vi "ziSetValueComplex.vi"(3 "Error In":errorcluster, 4 "Value":cdb, 5 "Path":string, 6 "Handle In":T1 {"Handle" format="0x%08x"; "Conn" format="0x%08x"}) -> (0 "Error Out":errorcluster, 2 "Handle Out":T1 {"Handle" format="0x%08x"; "Conn" format="0x%08x"})   [LabVIEW 2018, in "Zurich Instruments LabOne.lvlib"]
doc: "This vi sets values to the nodes specified in Path to Value. More than one node can be set if a wildcard is used in Path."
uses:
  Zurich Instruments LabOne.lvlib
  <instrlib>/Zurich Instruments LabOne/Private/ziLV64.framework
  ziTypeHandle.ctl
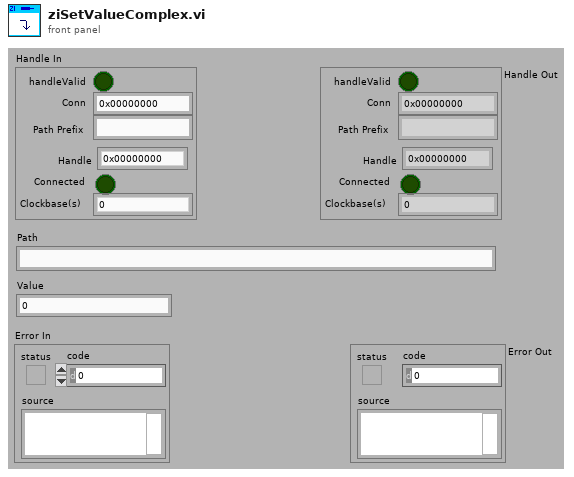
[diagram p1: front panel]
types:
  T1 = typedef "Zurich Instruments LabOne.lvlib/ziTypeHandle.ctl" = cluster{"handleValid":bool, "Conn":u64, "Path Prefix":string, "Handle":u64, "Connected":bool, "Clockbase(s)":dbl}
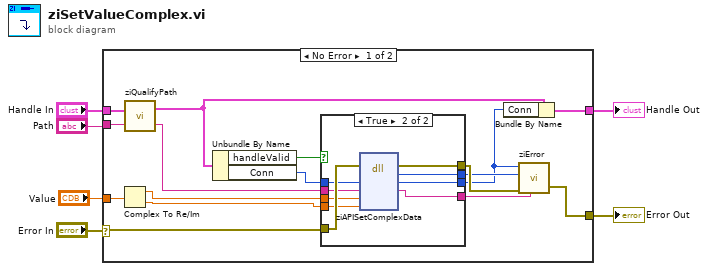
[diagram p0: block diagram]
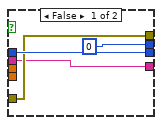
[diagram p2: hidden frame]
diagram:
  n1 = case shown="No Error" "Error In" {
    selector: "Error In" -> [w11 w37]
    tunnel: "Value" -> [w9 _]
    tunnel: [w21 w37] -> w5
    tunnel: [w17 w36] -> w4
    tunnel: "Handle In" -> [w16 w36]
    tunnel: "Path" -> [w14 _]
    frame No Error {
      n2 = Complex To Re/Im(x + iy=w9) -> (x=w8:dbl, y=w7:dbl)
      n3 = call "ziQualifyPath.vi"("Path In"=w14, "Handle In"=w16) -> ("Path Out"=w13:string, "Handle Out"=w15:T1)
      n4 = Unbundle By Name(w15) -> ("handleValid"=w18:bool, "Conn"=w22:u64)
      n5 = case shown="True" w18 {
        tunnel: w11 -> [w25 w35]
        tunnel: w22 -> [w26 w34]
        tunnel: w13 -> [w23 w33]
        tunnel: w8 -> [_ w32]
        tunnel: [w25 w31] -> w20
        tunnel: [u32 0 ("return type") w30] -> w19
        tunnel: [w26 w29] -> w10
        tunnel: [w23 w28] -> w12
        tunnel: w7 -> [_ w27]
        frame False {
        }
        frame True {
          n6 = dll-call lib="Applications/National Instruments/LabVIEW 2019 64-bit/instr.lib/Zurich Instruments LabOne/Private/ziLV*.*" fn="ziAPISetComplexData"(error in=w35, "Conn"=w34, "Path"=w33, "ValueR"=w32, "ValueI"=w27) -> (error out=w31:errorcluster, "return type"=w30:u32, "Conn"=w29:u64, "Path"=w28:string)  [unwired: 4 in, 1 out]
        }
      }
      n7 = Bundle By Name(cluster=w15, "Conn"=w10) -> (w17:T1)
      n8 = call "ziError.vi"("Conn"=w10, "ziErrorCode"=w19, "Error In"=w20, "Annotation"=w12) -> ("Error Out"=w21:errorcluster)  [unwired: 1 in, 1 out]
    }
    frame Error {
    }
  }
  "Error Out" <- w5
  "Handle Out" <- w4
